vi "OutputLayer.vi"(0 "OutputlayerIn":sgl[](array[numeric])=[0.0, 0.0]) -> (4 "OutputLayerOut":sgl)   [LabVIEW 2020]
uses:
  <vilib>/rvi/Memory/Memory_Emulation/nirvimemoryFastEmulation.vi
  <vilib>/rvi/Memory/Memory_Emulation/nirvimemoryEmulation.vi
  <vilib>/rvi/Emulation/niFpgaEmulationIsFPGAContextNoSignature.vi
  <vilib>/rvi/DataTransferAndStorage/Container/Common/niFpgaContainerGetUniqueNameForEmu.vi
  <vilib>/rvi/Emulation/niFpgaProcessEmulError.vi
  <vilib>/rvi/Emulation/niFpgaSctlEmulationGetInTimedLoop.vi
  <vilib>/rvi/errors/nirviReportUnexpectedCaseInternalError (U32).vi
  <vilib>/rvi/DataTransferAndStorage/Container/XNode/niFpgaContainer.xnode
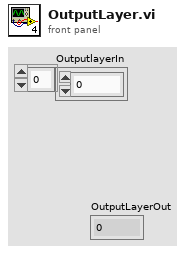
[diagram p1: front panel]
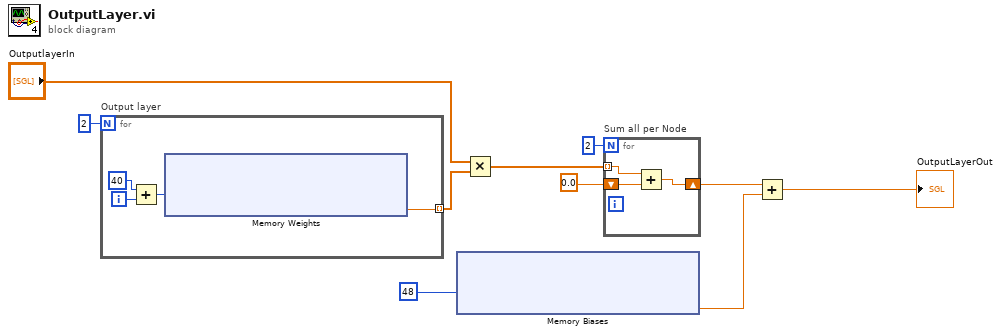
[diagram p0: block diagram]
diagram:
  n1 = for "Output layer" {
    N: 2 ("Size Previous layer") -> [_]
    tunnel: [w14] -> w8 mode=indexing
    i -> [w13]
    n2 = Add(x=40, y=w13) -> (x+y=w11:i32)
    n3 = xnode "Memory Weights"("Address"=w11) -> ("Data"=w14:sgl)  [unwired: 1 in, 1 out]
  }
  n4 = xnode "Memory Biases"("Address"=u32 48) -> ("Data"=w2:sgl)  [unwired: 1 in, 1 out]
  n5 = Multiply(x="OutputlayerIn", y=w8) -> (x*y=w1:sgl[])
  n6 = for "Sum all per Node" {
    N: 2 -> [_]
    tunnel: w1 -> [w17] mode=indexing
    shift-right: [w15] -> w3
    shift-left: sgl 0.0 -> [w16]
    n7 = Add(x=w17, y=w16) -> (x+y=w15:sgl)
  }
  n8 = Add(x=w3, y=w2) -> (x+y=→"OutputLayerOut":sgl)
